vi "Rotate Point.vi"(7 "Angle":dbl, 8 "Center Y":dbl, 9 "Center X":dbl, 10 "Y":dbl, 11 "X":dbl) -> (1 "Y":dbl, 3 "X":dbl)   [LabVIEW 2013]
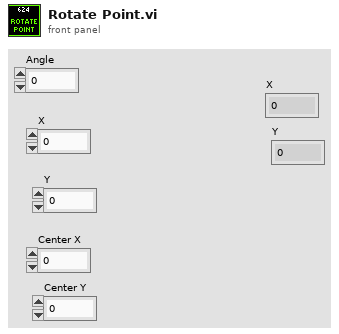
[diagram p1: front panel]
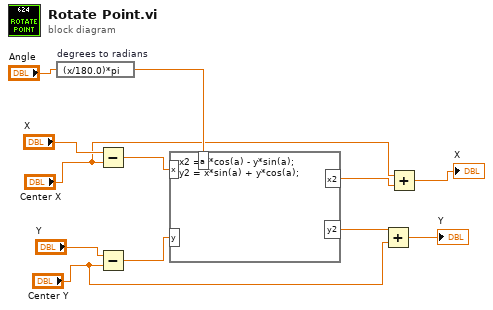
[diagram p0: block diagram]
diagram:
  n1 = expression code="(x/180.0)*pi" "degrees to radians"("Angle") -> (w7:dbl)
  n2 = Subtract(x="X", y="Center X") -> (x-y=w8:dbl)
  n3 = Subtract(x="Y", y="Center Y") -> (x-y=w9:dbl)
  n4 = formula code="x2 = x*cos(a) - y*sin(a);\ny2 = x*sin(a) + y*cos(a);"("x"=w8, "y"=w9, "a"=w7) -> ("x2"=w6:dbl, "y2"=w3:dbl)
  n5 = Add(x=w3, y="Center Y") -> (x+y=→"Y":dbl)
  n6 = Add(x="Center X", y=w6) -> (x+y=→"X":dbl)
